vi "Test Asic Rate Scan con tensiones.vi"(8 "Error IN":errorcluster, 11 "Config Test IN":T2={"Config HW"={"VISA Rigol DP832"="Rigol_DP832", "Config Rigol DP832"=[{"Channel"=0, "V Limit"=5.5, "I Limit"=0.5, "V Out"=5.0}, {"Channel"=1, "V Limit"=5.5, "I Limit"=0.8, "V Out"=5.0}, {"Channel"=2, "V Limit"=5.5, "I Limit"=0.2, "V Out"=0.0}], "CTA Test#"="CTA013 A", "FT_Handle"=0, "Espera acceso FT"=10, "VISA Tek MDO3104"="Rigol_DP832", "VISA Key 81160A"="Rigol_DP832"}, "Config Test"=[{"Vasic"=2.8, "Global Reset"=FALSE, "Test Register?"=FALSE, "Test ADC?"=FALSE, "Test ADC"={"Repeats ADC"=100, "Max Desviation"=0.1}, "Limits ADC"={"Low"=[1.9, 1.3, 0.65, 0.0, 1.6, 1.4, 1.4, 0.9, 2.1, 0.85, 1.9], "High"=[2.1, 1.5, 0.85, 0.1, 1.4, 1.2, 1.2, 0.7, 1.9, 0.65, 1.7]}, "Test Max PN Min NP?"=FALSE, "Limits Max PN Min NP"={"Max P Upper"=2.177000045776367, "Min P Upper"=1.474, "Max N Upper"=1.475, "Min N Upper"=0.818, "Max P Lower"=1.888, "Min P Lower "=1.321, "Max N Lower"=1.322, "Min N Lower"=0.73}, "Test Rate Scan?"=FALSE, "Vin Rate Scan"=[], "Limits Rate Scan"={"High"=[0.15, 0.242, 0.331, 0.425, 0.512, 0.6, 0.688, 0.774, 0.847, 0.91], "Low"=[0.021, 0.11, 0.189, 0.27, 0.347, 0.421, 0.487, 0.551, 0.601, 0.635]}, "Test Rate Scan Adders?"=FALSE, "Vin Rate Adders"=[], "Limits Rate Scan adders"={"High"=[], "Low"=[]}, "Test offset analog?"=FALSE, "Lim Offset Analog"={"Max Analog"=0.05, "Min Analog"=-0.05}, "Test offset digital?"=FALSE, "Lim offset Dig"={"Max Dig"=0.05}, "Vasic real f.a."=2.8, "IBIAS"=FALSE, "VALUE IBIAS"=63}, {"Vasic"=2.8, "Global Reset"=FALSE, "Test Register?"=FALSE, "Test ADC?"=FALSE, "Test ADC"={"Repeats ADC"=100, "Max Desviation"=0.1}, "Limits ADC"={"Low"=[1.9, 1.3, 0.65, 0.0, 1.6, 1.4, 1.4, 0.9, 2.1, 0.85, 1.9], "High"=[2.1, 1.5, 0.85, 0.1, 1.4, 1.2, 1.2, 0.7, 1.9, 0.65, 1.7]}, "Test Max PN Min NP?"=FALSE, "Limits Max PN Min NP"={"Max P Upper"=2.177000045776367, "Min P Upper"=1.474, "Max N Upper"=1.475, "Min N Upper"=0.818, "Max P Lower"=1.888, "Min P Lower "=1.321, "Max N Lower"=1.322, "Min N Lower"=0.73}, "Test Rate Scan?"=FALSE, "Vin Rate Scan"=[], "Limits Rate Scan"={"High"=[0.15, 0.242, 0.331, 0.425, 0.512, 0.6, 0.688, 0.774, 0.847, 0.91], "Low"=[0.021, 0.11, 0.189, 0.27, 0.347, 0.421, 0.487, 0.551, 0.601, 0.635]}, "Test Rate Scan Adders?"=FALSE, "Vin Rate Adders"=[], "Limits Rate Scan adders"={"High"=[], "Low"=[]}, "Test offset analog?"=FALSE, "Lim Offset Analog"={"Max Analog"=0.05, "Min Analog"=-0.05}, "Test offset digital?"=FALSE, "Lim offset Dig"={"Max Dig"=0.05}, "Vasic real f.a."=2.8, "IBIAS"=FALSE, "VALUE IBIAS"=63}, {"Vasic"=2.8, "Global Reset"=FALSE, "Test Register?"=FALSE, "Test ADC?"=FALSE, "Test ADC"={"Repeats ADC"=100, "Max Desviation"=0.1}, "Limits ADC"={"Low"=[1.9, 1.3, 0.65, 0.0, 1.6, 1.4, 1.4, 0.9, 2.1, 0.85, 1.9], "High"=[2.1, 1.5, 0.85, 0.1, 1.4, 1.2, 1.2, 0.7, 1.9, 0.65, 1.7]}, "Test Max PN Min NP?"=FALSE, "Limits Max PN Min NP"={"Max P Upper"=2.177000045776367, "Min P Upper"=1.474, "Max N Upper"=1.475, "Min N Upper"=0.818, "Max P Lower"=1.888, "Min P Lower "=1.321, "Max N Lower"=1.322, "Min N Lower"=0.73}, "Test Rate Scan?"=FALSE, "Vin Rate Scan"=[], "Limits Rate Scan"={"High"=[0.15, 0.242, 0.331, 0.425, 0.512, 0.6, 0.688, 0.774, 0.847, 0.91], "Low"=[0.021, 0.11, 0.189, 0.27, 0.347, 0.421, 0.487, 0.551, 0.601, 0.635]}, "Test Rate Scan Adders?"=FALSE, "Vin Rate Adders"=[], "Limits Rate Scan adders"={"High"=[], "Low"=[]}, "Test offset analog?"=FALSE, "Lim Offset Analog"={"Max Analog"=0.05, "Min Analog"=-0.05}, "Test offset digital?"=FALSE, "Lim offset Dig"={"Max Dig"=0.05}, "Vasic real f.a."=2.8, "IBIAS"=FALSE, "VALUE IBIAS"=63}, {"Vasic"=2.8, "Global Reset"=FALSE, "Test Register?"=FALSE, "Test ADC?"=FALSE, "Test ADC"={"Repeats ADC"=100, "Max Desviation"=0.1}, "Limits ADC"={"Low"=[1.9, 1.3, 0.65, 0.0, 1.6, 1.4, 1.4, 0.9, 2.1, 0.85, 1.9], "High"=[2.1, 1.5, 0.85, 0.1, 1.4, 1.2, 1.2, 0.7, 1.9, 0.65, 1.7]}, "Test Max PN Min NP?"=FALSE, "Limits Max PN Min NP"={"Max P Upper"=2.177000045776367, "Min P Upper"=1.474, "Max N Upper"=1.475, "Min N Upper"=0.818, "Max P Lower"=1.888, "Min P Lower "=1.321, "Max N Lower"=1.322, "Min N Lower"=0.73}, "Test Rate Scan?"=FALSE, "Vin Rate Scan"=[], "Limits Rate Scan"={"High"=[0.15, 0.242, 0.331, 0.425, 0.512, 0.6, 0.688, 0.774, 0.847, 0.91], "Low"=[0.021, 0.11, 0.189, 0.27, 0.347, 0.421, 0.487, 0.551, 0.601, 0.635]}, "Test Rate Scan Adders?"=FALSE, "Vin Rate Adders"=[], "Limits Rate Scan adders"={"High"=[], "Low"=[]}, "Test offset analog?"=FALSE, "Lim Offset Analog"={"Max Analog"=0.05, "Min Analog"=-0.05}, "Test offset digital?"=FALSE, "Lim offset Dig"={"Max Dig"=0.05}, "Vasic real f.a."=2.8, "IBIAS"=FALSE, "VALUE IBIAS"=63}], "Result"=[], "Execucion Test"={"Vasic Actual"=0}, "Config VGA"={"Theoretical Voltage"=[], "Real Voltage"=[102.85, 207.14, 299.57, 404.85, 495.71, 606.85, 697.71, 801.14, 897.14, 998.85], "Pulse Width"=57344, "Frecuency Pulse"=1000000.0, "VGA Gain"=[9, 16, 24, 34, 43, 52, 61, 72, 81, 93]}, "Test Info"={"Asic"="", "Operator"="", "Place"="", "Time start"=timestamp(0 s since 1904-01-01), "Time stop"=timestamp(0 s since 1904-01-01)}, "Info machine"={"SO"="", "SO Name"="", "SO Ver"="", "SO Build"="", "CPU"="", "APP"="", "APP YEAR"="", "APP ver"="", "APP User"="", "APP Serail"="", "MAC"=[], "PC NAME"=[], "PC IP"=[], "BIOS MANU"="", "BIOS NAME"="", "BIOS SERIAL"="", "BOARD MANU"="", "BOARD NAME"="", "BOARD SERIAL"="", "Driver Version"="", "Library Version"="", "FPGA Ver"=0, "ID CTA board"=0, "LAST BOOT"="", "LABVIEW Ver"=0}, "Partial Report"="", "CONFIG GEN"=[]} {"CONFIG GEN"."Vasic Theorical" min=1.0 max=1000000.0 step=1.0 format="%#_6pV"; "CONFIG GEN"."Frequency" min=0.001 max=333000000.0 step=1000.0 format="%#_6pHz"; "CONFIG GEN"."Leading Edge Time" min=1e-09 max=1.0 step=1e-10 format="%#_6ps"; "CONFIG GEN"."Trailing Edge Time" min=1e-09 max=1.0 step=1e-10 format="%#_6ps"; "CONFIG GEN"."Delay" min=0.0 max=1.0 step=1e-12 format="%#_6ps"; "CONFIG GEN"."Trigger Level Sync" items=["ECL", "TTL"]; "CONFIG GEN"."Trigger Sync Out" items=["AB"=3, "B"=2, "A"=1, "None"=0]; "CONFIG GEN"."Load" min=1.0 max=1000000.0 step=1.0 format="%#_6p"; "CONFIG GEN"."DC Offset" min=-10.0 max=10.0 step=0.1 format="%#_6pV"; "CONFIG GEN"."Amplitude" min=0.05 max=5.0 step=0.001 format="%#_6pV"; "CONFIG GEN"."Width Time" min=1.5e-09 max=1.0 step=1e-10 format="%#_6ps"; "CONFIG GEN"."Channel" items=["Channel1"=1, "Channel2"=2]; "Config VGA"."Theoretical Voltage" format="%1.4f"; "Config VGA"."VGA Gain" format="%02x"; "Config VGA"."Frecuency Pulse" format="%0_2p"; "Config VGA"."Pulse Width" format="%04x"; "Config VGA"."Real Voltage" format="%1.5f"; "Config Test"."VALUE IBIAS" max=63 step=1; "Config Test"."Vasic real f.a." min=2.8 max=3.8 step=0.01 format="%.2g"; "Config Test"."Limits Rate Scan adders"."Low" format="%1.3f"; "Config Test"."Limits Rate Scan adders"."High" format="%1.3f"; "Config Test"."Limits ADC"."High" format="%1.4f"; "Config Test"."Limits ADC"."Low" format="%1.3f"; "Config Test"."Lim offset Dig"."Max Dig" format="%.3g"; "Config Test"."Lim Offset Analog"."Min Analog" format="%.3g"; "Config Test"."Lim Offset Analog"."Max Analog" format="%.3g"; "Config Test"."Limits Rate Scan"."Low" format="%1.4f"; "Config Test"."Limits Rate Scan"."High" format="%1.3f"; "Config Test"."Limits Max PN Min NP"."Min P Upper" format="%.3g"; "Config Test"."Limits Max PN Min NP"."Min P Lower" format="%.3g"; "Config Test"."Limits Max PN Min NP"."Max N Lower" format="%.3g"; "Config Test"."Limits Max PN Min NP"."Max N Upper" format="%.3g"; "Config Test"."Limits Max PN Min NP"."Min N Lower" format="%.3g"; "Config Test"."Limits Max PN Min NP"."Min N Upper" format="%.3g"; "Config Test"."Limits Max PN Min NP"."Max P Upper" format="%.3g"; "Config Test"."Limits Max PN Min NP"."Max P Lower" format="%.3g"; "Config Test"."Vasic" min=2.8 max=3.8 step=0.01 format="%.2g"; "Config HW"."Config Rigol DP832"."Channel" items=["+30V Channel 1", "+30V Channel 2", "+5V Channel 3"]; "Config HW"."Config Rigol DP832"."V Limit" format="%.1g"; "Config HW"."Config Rigol DP832"."I Limit" format="%.1g"; "Config HW"."Config Rigol DP832"."V Out" format="%.1g"; "Result"."Test Registros"."Read W/R" format="%04x"; "Result"."Test Registros"."Pattern W/R" format="%04x"; "Result"."Test Registros"."Read Default" format="%04x"; "Result"."Test Registros"."Pattern Default" format="%04x"}) -> (0 "Error OUT":errorcluster, 2 "Rate scan all ok":bool, 3 "Config Test OUT":T2={"Config HW"={"VISA Rigol DP832"="Rigol_DP832", "Config Rigol DP832"=[{"Channel"=0, "V Limit"=5.5, "I Limit"=0.5, "V Out"=5.0}, {"Channel"=1, "V Limit"=5.5, "I Limit"=0.8, "V Out"=5.0}, {"Channel"=2, "V Limit"=5.5, "I Limit"=0.2, "V Out"=0.0}], "CTA Test#"="CTA013 A", "FT_Handle"=0, "Espera acceso FT"=10, "VISA Tek MDO3104"="Rigol_DP832", "VISA Key 81160A"="Rigol_DP832"}, "Config Test"=[{"Vasic"=2.8, "Global Reset"=FALSE, "Test Register?"=FALSE, "Test ADC?"=FALSE, "Test ADC"={"Repeats ADC"=100, "Max Desviation"=0.1}, "Limits ADC"={"Low"=[1.9, 1.3, 0.65, 0.0, 1.6, 1.4, 1.4, 0.9, 2.1, 0.85, 1.9], "High"=[2.1, 1.5, 0.85, 0.1, 1.4, 1.2, 1.2, 0.7, 1.9, 0.65, 1.7]}, "Test Max PN Min NP?"=FALSE, "Limits Max PN Min NP"={"Max P Upper"=2.177000045776367, "Min P Upper"=1.474, "Max N Upper"=1.475, "Min N Upper"=0.818, "Max P Lower"=1.888, "Min P Lower "=1.321, "Max N Lower"=1.322, "Min N Lower"=0.73}, "Test Rate Scan?"=FALSE, "Vin Rate Scan"=[], "Limits Rate Scan"={"High"=[0.15, 0.242, 0.331, 0.425, 0.512, 0.6, 0.688, 0.774, 0.847, 0.91], "Low"=[0.021, 0.11, 0.189, 0.27, 0.347, 0.421, 0.487, 0.551, 0.601, 0.635]}, "Test Rate Scan Adders?"=FALSE, "Vin Rate Adders"=[], "Limits Rate Scan adders"={"High"=[], "Low"=[]}, "Test offset analog?"=FALSE, "Lim Offset Analog"={"Max Analog"=0.05, "Min Analog"=-0.05}, "Test offset digital?"=FALSE, "Lim offset Dig"={"Max Dig"=0.05}, "Vasic real f.a."=2.8, "IBIAS"=FALSE, "VALUE IBIAS"=63}, {"Vasic"=2.8, "Global Reset"=FALSE, "Test Register?"=FALSE, "Test ADC?"=FALSE, "Test ADC"={"Repeats ADC"=100, "Max Desviation"=0.1}, "Limits ADC"={"Low"=[1.9, 1.3, 0.65, 0.0, 1.6, 1.4, 1.4, 0.9, 2.1, 0.85, 1.9], "High"=[2.1, 1.5, 0.85, 0.1, 1.4, 1.2, 1.2, 0.7, 1.9, 0.65, 1.7]}, "Test Max PN Min NP?"=FALSE, "Limits Max PN Min NP"={"Max P Upper"=2.177000045776367, "Min P Upper"=1.474, "Max N Upper"=1.475, "Min N Upper"=0.818, "Max P Lower"=1.888, "Min P Lower "=1.321, "Max N Lower"=1.322, "Min N Lower"=0.73}, "Test Rate Scan?"=FALSE, "Vin Rate Scan"=[], "Limits Rate Scan"={"High"=[0.15, 0.242, 0.331, 0.425, 0.512, 0.6, 0.688, 0.774, 0.847, 0.91], "Low"=[0.021, 0.11, 0.189, 0.27, 0.347, 0.421, 0.487, 0.551, 0.601, 0.635]}, "Test Rate Scan Adders?"=FALSE, "Vin Rate Adders"=[], "Limits Rate Scan adders"={"High"=[], "Low"=[]}, "Test offset analog?"=FALSE, "Lim Offset Analog"={"Max Analog"=0.05, "Min Analog"=-0.05}, "Test offset digital?"=FALSE, "Lim offset Dig"={"Max Dig"=0.05}, "Vasic real f.a."=2.8, "IBIAS"=FALSE, "VALUE IBIAS"=63}, {"Vasic"=2.8, "Global Reset"=FALSE, "Test Register?"=FALSE, "Test ADC?"=FALSE, "Test ADC"={"Repeats ADC"=100, "Max Desviation"=0.1}, "Limits ADC"={"Low"=[1.9, 1.3, 0.65, 0.0, 1.6, 1.4, 1.4, 0.9, 2.1, 0.85, 1.9], "High"=[2.1, 1.5, 0.85, 0.1, 1.4, 1.2, 1.2, 0.7, 1.9, 0.65, 1.7]}, "Test Max PN Min NP?"=FALSE, "Limits Max PN Min NP"={"Max P Upper"=2.177000045776367, "Min P Upper"=1.474, "Max N Upper"=1.475, "Min N Upper"=0.818, "Max P Lower"=1.888, "Min P Lower "=1.321, "Max N Lower"=1.322, "Min N Lower"=0.73}, "Test Rate Scan?"=FALSE, "Vin Rate Scan"=[], "Limits Rate Scan"={"High"=[0.15, 0.242, 0.331, 0.425, 0.512, 0.6, 0.688, 0.774, 0.847, 0.91], "Low"=[0.021, 0.11, 0.189, 0.27, 0.347, 0.421, 0.487, 0.551, 0.601, 0.635]}, "Test Rate Scan Adders?"=FALSE, "Vin Rate Adders"=[], "Limits Rate Scan adders"={"High"=[], "Low"=[]}, "Test offset analog?"=FALSE, "Lim Offset Analog"={"Max Analog"=0.05, "Min Analog"=-0.05}, "Test offset digital?"=FALSE, "Lim offset Dig"={"Max Dig"=0.05}, "Vasic real f.a."=2.8, "IBIAS"=FALSE, "VALUE IBIAS"=63}, {"Vasic"=2.8, "Global Reset"=FALSE, "Test Register?"=FALSE, "Test ADC?"=FALSE, "Test ADC"={"Repeats ADC"=100, "Max Desviation"=0.1}, "Limits ADC"={"Low"=[1.9, 1.3, 0.65, 0.0, 1.6, 1.4, 1.4, 0.9, 2.1, 0.85, 1.9], "High"=[2.1, 1.5, 0.85, 0.1, 1.4, 1.2, 1.2, 0.7, 1.9, 0.65, 1.7]}, "Test Max PN Min NP?"=FALSE, "Limits Max PN Min NP"={"Max P Upper"=2.177000045776367, "Min P Upper"=1.474, "Max N Upper"=1.475, "Min N Upper"=0.818, "Max P Lower"=1.888, "Min P Lower "=1.321, "Max N Lower"=1.322, "Min N Lower"=0.73}, "Test Rate Scan?"=FALSE, "Vin Rate Scan"=[], "Limits Rate Scan"={"High"=[0.15, 0.242, 0.331, 0.425, 0.512, 0.6, 0.688, 0.774, 0.847, 0.91], "Low"=[0.021, 0.11, 0.189, 0.27, 0.347, 0.421, 0.487, 0.551, 0.601, 0.635]}, "Test Rate Scan Adders?"=FALSE, "Vin Rate Adders"=[], "Limits Rate Scan adders"={"High"=[], "Low"=[]}, "Test offset analog?"=FALSE, "Lim Offset Analog"={"Max Analog"=0.05, "Min Analog"=-0.05}, "Test offset digital?"=FALSE, "Lim offset Dig"={"Max Dig"=0.05}, "Vasic real f.a."=2.8, "IBIAS"=FALSE, "VALUE IBIAS"=63}], "Result"=[], "Execucion Test"={"Vasic Actual"=0}, "Config VGA"={"Theoretical Voltage"=[], "Real Voltage"=[102.85, 207.14, 299.57, 404.85, 495.71, 606.85, 697.71, 801.14, 897.14, 998.85], "Pulse Width"=57344, "Frecuency Pulse"=1000000.0, "VGA Gain"=[9, 16, 24, 34, 43, 52, 61, 72, 81, 93]}, "Test Info"={"Asic"="", "Operator"="", "Place"="", "Time start"=timestamp(0 s since 1904-01-01), "Time stop"=timestamp(0 s since 1904-01-01)}, "Info machine"={"SO"="", "SO Name"="", "SO Ver"="", "SO Build"="", "CPU"="", "APP"="", "APP YEAR"="", "APP ver"="", "APP User"="", "APP Serail"="", "MAC"=[], "PC NAME"=[], "PC IP"=[], "BIOS MANU"="", "BIOS NAME"="", "BIOS SERIAL"="", "BOARD MANU"="", "BOARD NAME"="", "BOARD SERIAL"="", "Driver Version"="", "Library Version"="", "FPGA Ver"=0, "ID CTA board"=0, "LAST BOOT"="", "LABVIEW Ver"=0}, "Partial Report"="", "CONFIG GEN"=[]} {"CONFIG GEN"."Vasic Theorical" min=1.0 max=1000000.0 step=1.0 format="%#_6pV"; "CONFIG GEN"."Frequency" min=0.001 max=333000000.0 step=1000.0 format="%#_6pHz"; "CONFIG GEN"."Leading Edge Time" min=1e-09 max=1.0 step=1e-10 format="%#_6ps"; "CONFIG GEN"."Trailing Edge Time" min=1e-09 max=1.0 step=1e-10 format="%#_6ps"; "CONFIG GEN"."Delay" min=0.0 max=1.0 step=1e-12 format="%#_6ps"; "CONFIG GEN"."Trigger Level Sync" items=["ECL", "TTL"]; "CONFIG GEN"."Trigger Sync Out" items=["AB"=3, "B"=2, "A"=1, "None"=0]; "CONFIG GEN"."Load" min=1.0 max=1000000.0 step=1.0 format="%#_6p"; "CONFIG GEN"."DC Offset" min=-10.0 max=10.0 step=0.1 format="%#_6pV"; "CONFIG GEN"."Amplitude" min=0.05 max=5.0 step=0.001 format="%#_6pV"; "CONFIG GEN"."Width Time" min=1.5e-09 max=1.0 step=1e-10 format="%#_6ps"; "CONFIG GEN"."Channel" items=["Channel1"=1, "Channel2"=2]; "Config VGA"."Theoretical Voltage" format="%1.4f"; "Config VGA"."VGA Gain" format="%02x"; "Config VGA"."Frecuency Pulse" format="%0_2p"; "Config VGA"."Pulse Width" format="%04x"; "Config VGA"."Real Voltage" format="%1.5f"; "Config Test"."VALUE IBIAS" max=63 step=1; "Config Test"."Vasic real f.a." min=2.8 max=3.8 step=0.01 format="%.2g"; "Config Test"."Limits Rate Scan adders"."Low" format="%1.3f"; "Config Test"."Limits Rate Scan adders"."High" format="%1.3f"; "Config Test"."Limits ADC"."High" format="%1.4f"; "Config Test"."Limits ADC"."Low" format="%1.3f"; "Config Test"."Lim offset Dig"."Max Dig" format="%.3g"; "Config Test"."Lim Offset Analog"."Min Analog" format="%.3g"; "Config Test"."Lim Offset Analog"."Max Analog" format="%.3g"; "Config Test"."Limits Rate Scan"."Low" format="%1.4f"; "Config Test"."Limits Rate Scan"."High" format="%1.3f"; "Config Test"."Limits Max PN Min NP"."Min P Upper" format="%.3g"; "Config Test"."Limits Max PN Min NP"."Min P Lower" format="%.3g"; "Config Test"."Limits Max PN Min NP"."Max N Lower" format="%.3g"; "Config Test"."Limits Max PN Min NP"."Max N Upper" format="%.3g"; "Config Test"."Limits Max PN Min NP"."Min N Lower" format="%.3g"; "Config Test"."Limits Max PN Min NP"."Min N Upper" format="%.3g"; "Config Test"."Limits Max PN Min NP"."Max P Upper" format="%.3g"; "Config Test"."Limits Max PN Min NP"."Max P Lower" format="%.3g"; "Config Test"."Vasic" min=2.8 max=3.8 step=0.01 format="%.2g"; "Config HW"."Config Rigol DP832"."Channel" items=["+30V Channel 1", "+30V Channel 2", "+5V Channel 3"]; "Config HW"."Config Rigol DP832"."V Limit" format="%.1g"; "Config HW"."Config Rigol DP832"."I Limit" format="%.1g"; "Config HW"."Config Rigol DP832"."V Out" format="%.1g"; "Result"."Test Registros"."Read W/R" format="%04x"; "Result"."Test Registros"."Pattern W/R" format="%04x"; "Result"."Test Registros"."Read Default" format="%04x"; "Result"."Test Registros"."Pattern Default" format="%04x"})   [LabVIEW 2019]
uses:
  Test.ctl
  TEST.TEST CONFIG HW.ctl
  Rigol DP832/DP832_Control Channels.ctl
  TEST.TEST CONFIG TEST MATRIZ.ctl
  TEST.TEST CONFIG TEST.ctl
  TEST.TEST RESULT.ctl
  test_result fvasic.ctl
  TEST.TEST EXECUTION TEST.ctl
  TEST.TEST CONFIG VGA.ctl
  TEST.TEST TEST INFO.ctl
  TEST.TEST INFO PC.ctl
  GenPulse_configurar.ctl
  Global.Salir Ya.vi
panel:
  out "Array 2":dbl[](array[numeric])
  out "Array":dbl[](array[numeric])
  in  "DAC\nTH0,TH1,TH2":u16
  in  "Tab Control":enum32{"Page 1", "Page 2"}(tab)
  out "%":u8 format="%02d%%"
  out "B":u8(slide) scale=0.0..100.0
  out "Indicador":string
  out "Comparation LLTH":bool[][][](array[boolean])
  out "Comparation HLTH":bool[][][](array[boolean])
  out "Reference":T1
  out "DAC TH3,TH4,TH5":u16
  out "LLTHx":dbl
  out "DAC TH0,TH1,TH2":u16
  out "HLTHx":dbl
  out "Volt LLTH (salida B)":dbl[][][](array[numeric])
  out "Volt HLTH (salida A)":dbl[][][](array[numeric])
  out "DAC TH3,TH4,TH5":u16[][][](array[numeric])
  out "DAC TH0,TH1,TH2":u16[][][](array[numeric])
  # "Vin Asic"
  # "Canal"
  # "Sumador"
  # "Test ASIC. Rate Scan"
  # "Modo 2\nModo 3\nModo 4\nModo 2\nModo 3\nModo 4"
  # "Modo 2\nModo 3\nModo 4\nModo 2\nModo 3\nModo 4"
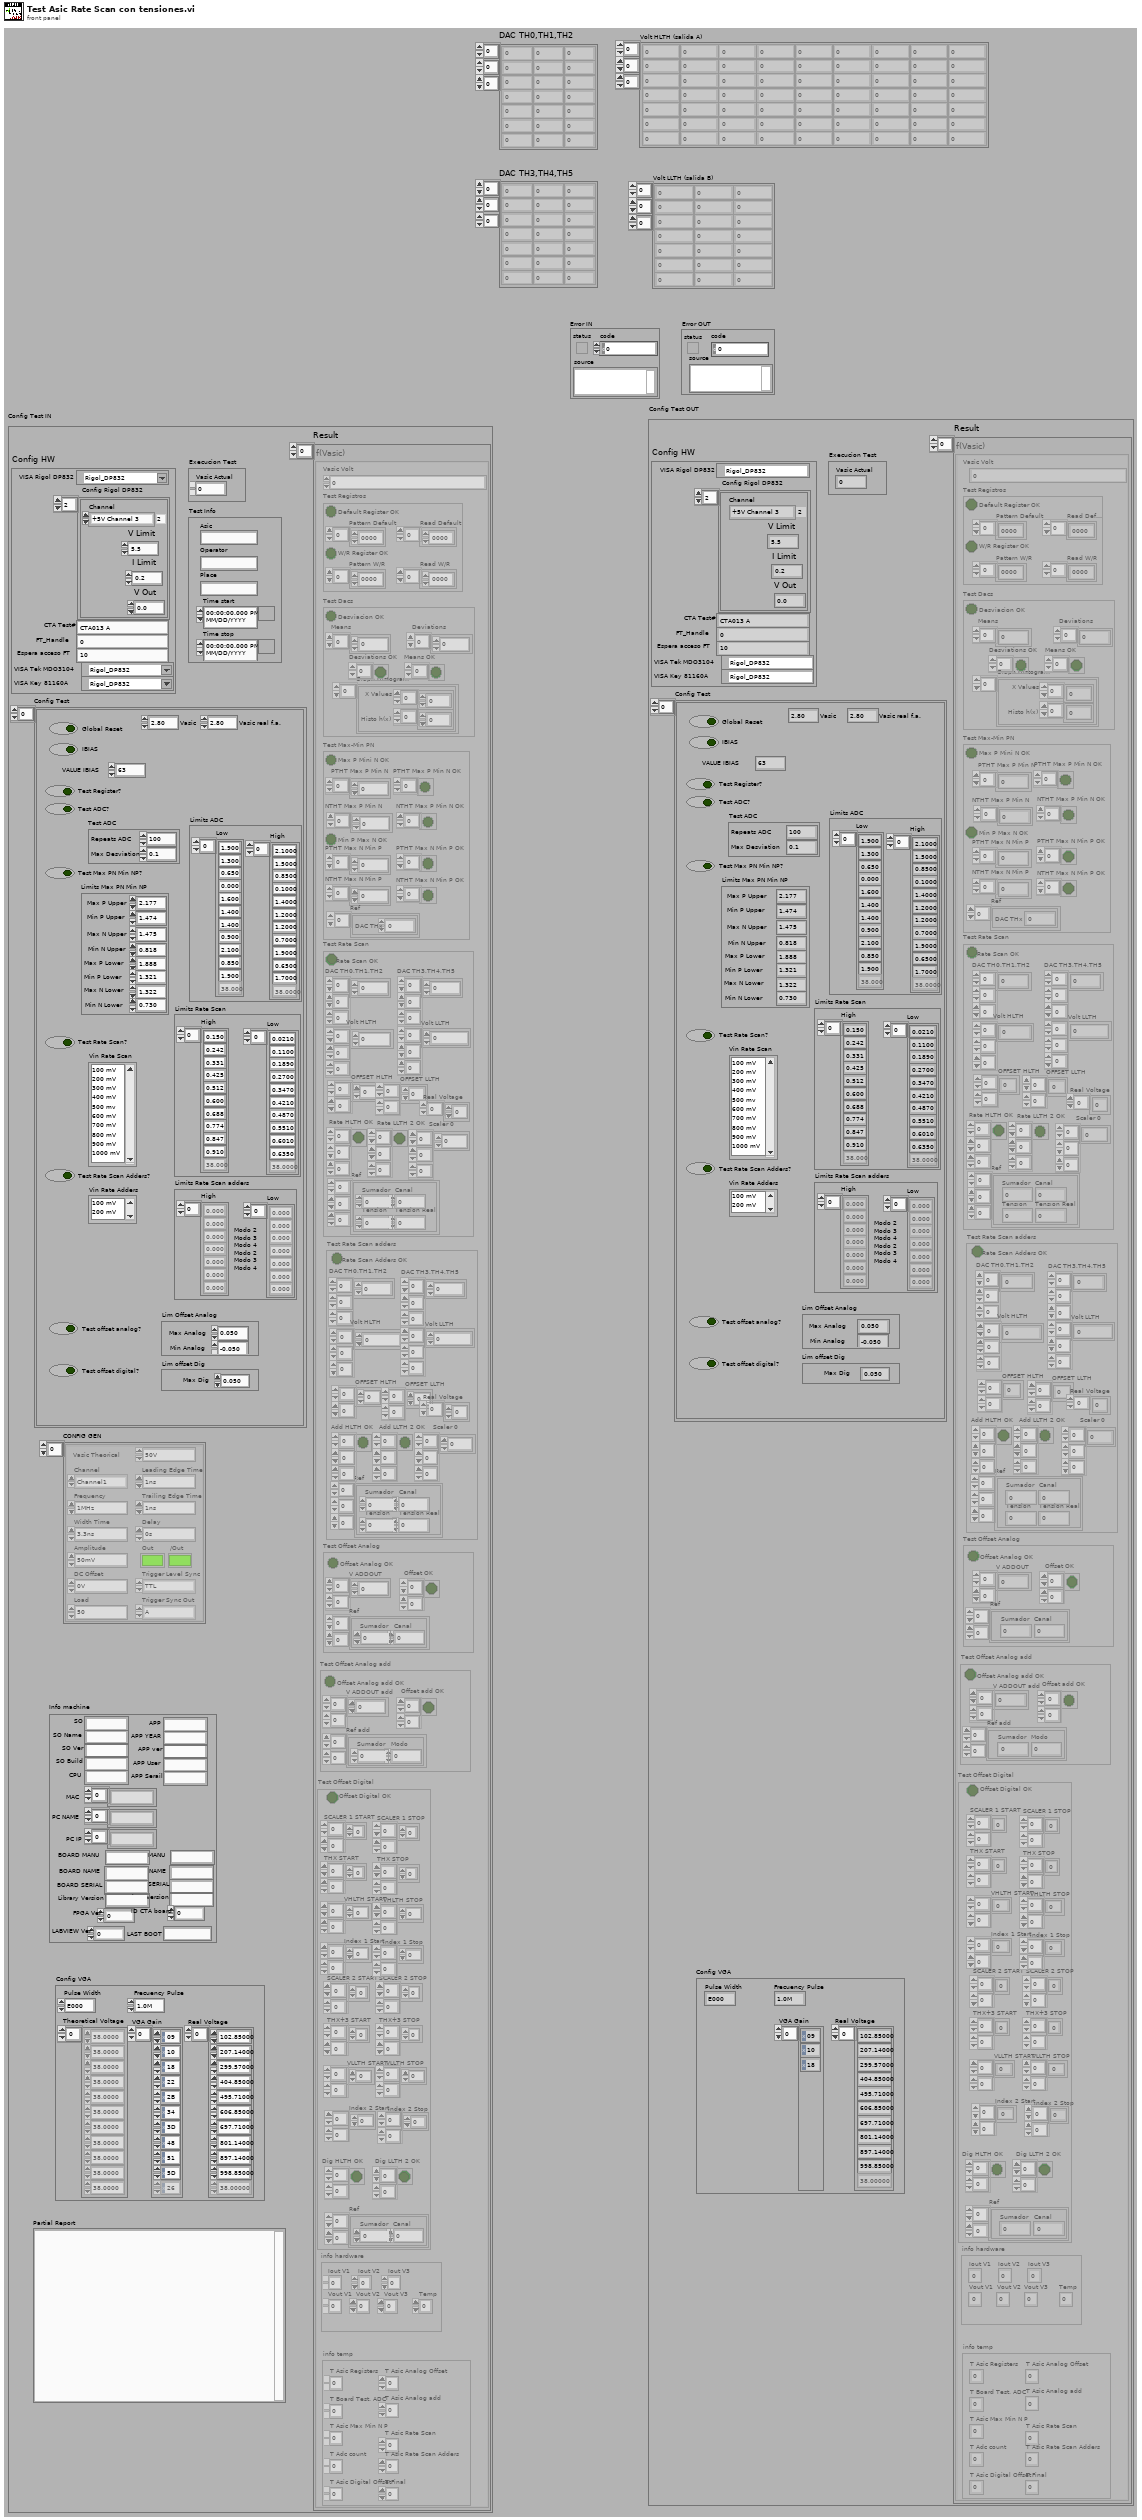
[diagram p1: front panel]
types:
  T1 = cluster{"Sumador":u8, "Canal":u8, "Tension":u8, "Tension Real":dbl}
  T2 = typedef "Test.ctl" = cluster{"Config HW":T3, "Config Test":T5, "Result":T7, "Execucion Test":T9, "Config VGA":T10, "Test Info":T11, "Info machine":T12, "Partial Report":string, "CONFIG GEN":T13[]}
  T3 = typedef "TEST.TEST CONFIG HW.ctl" = cluster{"VISA Rigol DP832":refnum<visa-resource-name>, "Config Rigol DP832":cluster{"Channel":T4, "V Limit":dbl, "I Limit":dbl, "V Out":dbl}[], "CTA Test#":string, "FT_Handle":u32, "Espera acceso FT":u32, "VISA Tek MDO3104":refnum<visa-resource-name>, "VISA Key 81160A":refnum<visa-resource-name>}
  T4 = typedef "DP832_Control Channels.ctl" = i32
  T5 = typedef "TEST.TEST CONFIG TEST MATRIZ.ctl" = T6[]
  T6 = typedef "TEST.TEST CONFIG TEST.ctl" = cluster{"Vasic":dbl, "Global Reset":bool, "Test Register?":bool, "Test ADC?":bool, "Test ADC":cluster{"Repeats ADC":i32, "Max Desviation":dbl}, "Limits ADC":cluster{"Low":dbl[], "High":dbl[]}, "Test Max PN Min NP?":bool, "Limits Max PN Min NP":cluster{"Max P Upper":dbl, "Min P Upper":dbl, "Max N Upper":dbl, "Min N Upper":dbl, "Max P Lower":dbl, "Min P Lower ":dbl, "Max N Lower":dbl, "Min N Lower":dbl}, "Test Rate Scan?":bool, "Vin Rate Scan":i32[], "Limits Rate Scan":cluster{"High":dbl[], "Low":dbl[]}, "Test Rate Scan Adders?":bool, "Vin Rate Adders":i32[], "Limits Rate Scan adders":cluster{"High":dbl[], "Low":dbl[]}, "Test offset analog?":bool, "Lim Offset Analog":cluster{"Max Analog":dbl, "Min Analog":dbl}, "Test offset digital?":bool, "Lim offset Dig":cluster{"Max Dig":dbl}, "Vasic real f.a.":dbl, "IBIAS":bool, "VALUE IBIAS":u8}
  T7 = typedef "TEST.TEST RESULT.ctl" = T8[]
  T8 = typedef "test_result fvasic.ctl" = cluster{"Vasic Volt":i32, "Test Registros":cluster{"Default Register OK":bool, "Pattern Default":u16[], "Read Default":u16[], "W/R Register OK":bool, "Pattern W/R":u16[], "Read W/R":u16[]}, "Test Dacs":cluster{"Desviacion OK":bool, "Means":dbl[], "Deviations":dbl[], "Desviations OK":bool[], "Means OK":bool[], "Graph Histogram":cluster{"X Values":dbl[], "Histo h(x)":i32[]}[]}, "Test Max-Min PN":cluster{"Max P Mini N OK":bool, "PTHT Max P Min N":dbl[], "PTHT Max P Min N OK":bool[], "NTHT Max P Min N":dbl[], "NTHT Max P Min N OK":bool[], "Min P Max N OK":bool, "PTHT Max N Min P":dbl[], "PTHT Max N Min P OK":bool[], "NTHT Max N Min P":dbl[], "NTHT Max N Min P OK":bool[], "Ref":cluster{"DAC THx":u8}[]}, "Test Rate Scan":cluster{"Rate Scan OK":bool, "DAC TH0,TH1,TH2":u16[][][], "Volt HLTH":dbl[][][], "Rate HLTH OK":bool[][][], "DAC TH3,TH4,TH5":u16[][][], "Volt LLTH":dbl[][][], "Rate LLTH 2 OK":bool[][][], "Scaler 0":u16[][][], "Ref":cluster{"Sumador":u8, "Canal":u8, "Tension":u8, "Tension Real":dbl}[][][], "OFFSET HLTH":dbl[][], "OFFSET LLTH":dbl[][], "Real Voltage":dbl[]}, "Test Rate Scan adders":cluster{"Rate Scan Adders OK":bool, "DAC TH0,TH1,TH2":u16[][][], "Volt HLTH":dbl[][][], "Add HLTH OK":bool[][][], "DAC TH3,TH4,TH5":u16[][][], "Volt LLTH":dbl[][][], "Add LLTH 2 OK":bool[][][], "Scaler 0":u16[][][], "Ref":cluster{"Sumador":u8, "Canal":u8, "Tension":u8, "Tension Real":dbl}[][][], "OFFSET HLTH":dbl[][], "OFFSET LLTH":dbl[][], "Real Voltage":dbl[]}, "Test Offset Analog":cluster{"Offset Analog OK":bool, "V ADDOUT":dbl[][], "Offset OK":bool[][], "Ref":cluster{"Sumador":u8, "Canal":u8}[][]}, "Test Offset Digital":cluster{"Offset Digital OK":bool, "SCALER 1 START":u16[][], "SCALER 1 STOP":u16[][], "THX START":u16[][], "THX STOP":u16[][], "VHLTH START":dbl[][], "VHLTH STOP":dbl[][], "Index 1 Start":i32[][], "index 1 Stop":i32[][], "SCALER 2 START":u16[][], "SCALER 2 STOP":u16[][], "THX+3 START":u16[][], "THX+3 STOP":u16[][], "VLLTH START":dbl[][], "VLLTH STOP":dbl[][], "Index 2 Start":i32[][], "index 2 Stop":i32[][], "Dig HLTH OK":bool[][], "Dig LLTH 2 OK":bool[][], "Ref":cluster{"Sumador":u8, "Canal":u8}[][]}, "info hardware":cluster{"Iout V1":dbl, "Iout V2":dbl, "Iout V3":dbl, "Vout V1":dbl, "Vout V2":dbl, "Vout V3":dbl, "Temp":dbl}, "Test Offset Analog add":cluster{"Offset Analog add OK":bool, "V ADDOUT add":dbl[][], "Offset add OK":bool[][], "Ref add":cluster{"Sumador":u8, "Modo":u8}[][]}, "info temp":cluster{"T Asic Registers":dbl, "T Board Test. ADC":dbl, "T Asic Max Min N P":dbl, "T Adc count":dbl, "T Asic Digital Offset":dbl, "T Asic Analog Offset":dbl, "T Asic Analog add":dbl, "T Asic Rate Scan":dbl, "T Asic Rate Scan Adders":dbl, "T Final":dbl}}
  T9 = typedef "TEST.TEST EXECUTION TEST.ctl" = cluster{"Vasic Actual":i32}
  T10 = typedef "TEST.TEST CONFIG VGA.ctl" = cluster{"Theoretical Voltage":dbl[], "Real Voltage":dbl[], "Pulse Width":u16, "Frecuency Pulse":dbl, "VGA Gain":u8[]}
  T11 = typedef "TEST.TEST TEST INFO.ctl" = cluster{"Asic":string, "Operator":string, "Place":string, "Time start":timestamp, "Time stop":timestamp}
  T12 = typedef "TEST.TEST INFO PC.ctl" = cluster{"SO":string, "SO Name":string, "SO Ver":string, "SO Build":string, "CPU":string, "APP":string, "APP YEAR":string, "APP ver":string, "APP User":string, "APP Serail":string, "MAC":string[], "PC NAME":string[], "PC IP":string[], "BIOS MANU":string, "BIOS NAME":string, "BIOS SERIAL":string, "BOARD MANU":string, "BOARD NAME":string, "BOARD SERIAL":string, "Driver Version":string, "Library Version":string, "FPGA Ver":u8, "ID CTA board":u64, "LAST BOOT":string, "LABVIEW Ver":u32}
  T13 = typedef "GenPulse_configurar.ctl" = cluster{"Channel":u16, "Frequency":dbl, "Width Time":dbl, "Amplitude":dbl, "DC Offset":dbl, "Load":dbl, "Leading Edge Time":dbl, "Trailing Edge Time":dbl, "Delay":dbl, "Out":bool, "/Out":bool, "Trigger Level Sync":u16, "Trigger Sync Out":u16, "Vasic Theorical":dbl}
  T14 = enum16{"Always On", "Always Off", "Off While Running"}
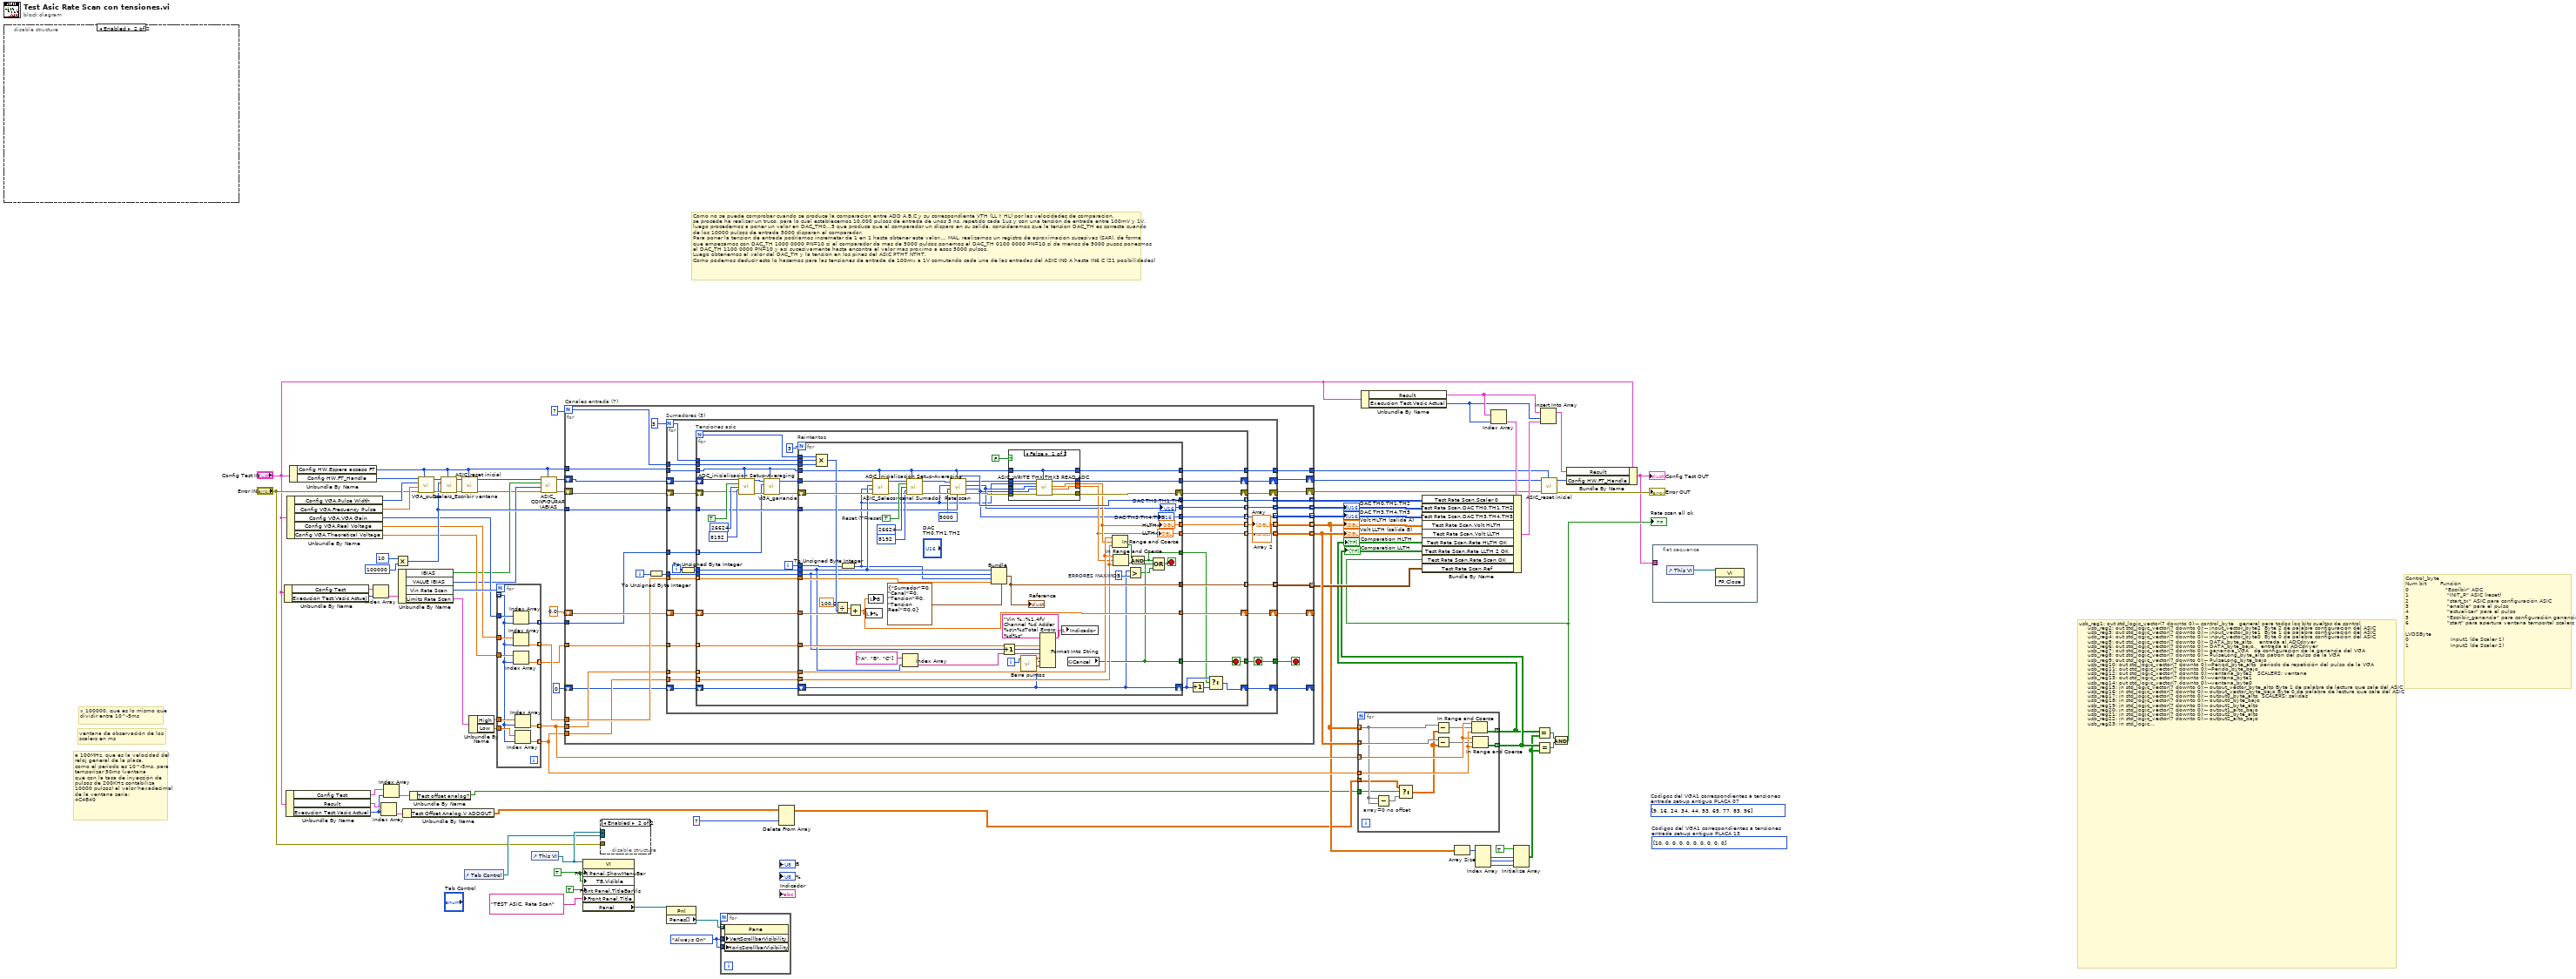
[diagram p0: block diagram]
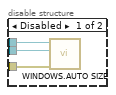
[diagram p2: hidden frame]
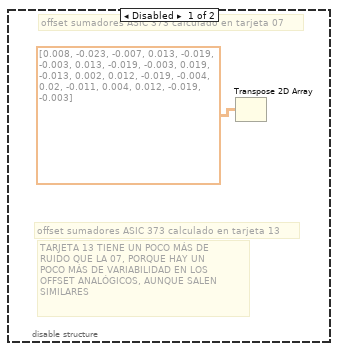
[diagram p3: hidden frame]
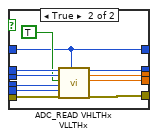
[diagram p4: hidden frame]
diagram:
  w1 = T14."Always On" ("Vertical Scrollbar Visibility")
  w35 = TRUE ("Front Panel Window:Show Menu Bar")
  (unwired) u8[] [10, 0, 0, 0, 0, 0, 0, 0, 0, 0]  # Códigos del VGA1 correspondientes a tensiones entrada set-up antiguo PLACA 13
  (unwired) u8[] [9, 16, 24, 34, 44, 53, 65, 77, 83, 96]  # Códigos del VGA1 correspondientes a tensiones entrada set-up antiguo PLACA 07
  # "Como no se puede comprobar cuando se produce la comparacion entre ADD A,B,C y su correspondiente VTH (LL Y HL) por las velocidades de comparacion,\nse procede ha realizar un truco, para lo cual establecemos 10.000 pulsos de entrada de unos 3 ns, repetido cada 1us y con una tension de entrada entre 100mV y 1V,\nluego procedemos a poner un valor en DAC_TH0...5 que produca que el comparador un disparo en su salida, consideramos que la tension DAC_TH es correcta cuando\nde los 10000 pulsos de entrada 5000 disparan el comparador.\nPara poner la tension de entrada podriamos incremetar de 1 en 1 hasta obtener este valor.... MAL. realizamos un registro de aproximacion sucesivas (SAR), de forma\nque empezamos con DAC_TH 1000 0000 PN=10 si el comparador da mas de 5000 pulsos ponemos el DAC_TH 0100 0000 PN=10 si da menos de 5000 pusos ponesmos\nel DAC_TH 1100 0000 PN=10 y asi sucesivamente hasta encontra el valor mas proximo a esos 5000 pulsos. \nLuego obtenemos el valor del DAC_TH y la tension en los pines del ASIC PTHT NTHT.\nComo podemos deducir esto lo hacemos para las tensiones de entrada de 100mv a 1V comutando cada una de las entradas del ASIC IN0 A hasta IN6 C (21 posibilidades)"
  # "Control_byte\nNum bit        Función\n0                     \"Escribir\" ADC\n1                      \"INIT_R\" ASIC (reset)\n2                      \"start_tx\" ASIC para configuración ASIC\n3                      \"enable\" para el pulso\n4                      \"actualizar\" para el pulso\n5                      \"Escribir_ganancia\" para configuración ganancia\n6                      \"start\" para apertura ventana temportal scalers\n\nLVDSByte\n0                        Input1 (de Scaler 1)\n1                        Input2 (de Scaler 2)"
  # "usb_reg1: out std_logic_vector(7 downto 0);-- control_byte\t\t\tgeneral para todos los bits sueltos de control\n\t\t\t  usb_reg2: out std_logic_vector(7 downto 0);-- input_vector_byte2 \tByte 2 de palabra configuración del ASIC\n\t\t\t  usb_reg3: out std_logic_vector(7 downto 0);-- input_vector_byte1 \tByte 1 de palabra configuración del ASIC\n\t\t\t  usb_reg4: out std_logic_vector(7 downto 0);-- input_vector_byte0 \tByte 0 de palabra configuración del ASIC\n\t\t\t  usb_reg5: out std_logic_vector(7 downto 0);-- DATA_byte_alto, \t\tentrada al ADCdriver\n\t\t\t  usb_reg6: out std_logic_vector(7 downto 0);-- DATA_byte_bajo, \t\tentrada al ADCdriver\n\t\t\t  usb_reg7: out std_logic_vector(7 downto 0);-- ganancia_VGA\t\t\tde configuración de la ganancia del VGA\n\t\t\t  usb_reg8: out std_logic_vector(7 downto 0);-- PulseLong_byte_alto\tpatrón del pulso de la VGA\n\t\t\t  usb_reg9: out std_logic_vector(7 downto 0);-- PulseLong_byte_bajo\n\t\t\t  usb_reg10: out std_logic_vector(7 downto 0);--Period_byte_alto\t\tperíodo de repetición del pulso de la VGA\n\t\t\t  usb_reg11: out std_logic_vector(7 downto 0);--Perido_byte_bajo\n\t\t\t  usb_reg12: out std_logic_vector(7 downto 0);--ventana_byte2\t\t\tSCALERS: ventana\n\t\t\t  usb_reg13: out std_logic_vector(7 downto 0);--ventana_byte1\t\n\t\t\t  usb_reg14: out std_logic_vector(7 downto 0);--ventana_byte0\n\t\t\t  usb_reg15: in std_logic_vector(7 downto 0);-- output_vector_byte_alto\tByte 1 de palabra de lectura que sale del ASIC\n\t\t\t  usb_reg16: in std_logic_vector(7 downto 0);-- output_vector_byte_bajo\tByte 0 de palabra de lectura que sale del ASIC\n\t\t\t  usb_reg17: in std_logic_vector(7 downto 0);-- output0_byte_alto\t\tSCALERS: salidas\n\t\t\t  usb_reg18: in std_logic_vector(7 downto 0);-- output0_byte_bajo\n\t\t\t  usb_reg19: in std_logic_vector(7 downto 0);-- output1_byte_alto\n\t\t\t  usb_reg20: in std_logic_vector(7 downto 0);-- output1_alto_bajo \n\t\t\t  usb_reg21: in std_logic_vector(7 downto 0);-- output2_byte_alto \n\t\t\t  usb_reg22: in std_logic_vector(7 downto 0);-- output2_alto_bajo \n\t\t\t  usb_reg23: in std_logic_vector(7 downto 0);-- para el canal_0 del ADCdriver\n\t\t\t  usb_reg24: in std_logic_vector(7 downto 0);\n\t\t\t  usb_reg25: in std_logic_vector(7 downto 0);-- para el canal_1 del ADCdriver\n\t\t\t  usb_reg26: in std_logic_vector(7 downto 0);\n\t\t\t  usb_reg27: in std_logic_vector(7 downto 0);-- para el canal_2 del ADCdriver\n\t\t\t  usb_reg28: in std_logic_vector(7 downto 0);\n\t\t\t  usb_reg29: in std_logic_vector(7 downto 0);-- para el canal_3 del ADCdriver\n\t\t\t  usb_reg30: in std_logic_vector(7 downto 0);\n\t\t\t  usb_reg31: in std_logic_vector(7 downto 0);-- para el canal_4 del ADCdriver\n\t\t\t  usb_reg32: in std_logic_vector(7 downto 0);\n\t\t\t  usb_reg33: in std_logic_vector(7 downto 0);-- para el canal_5 del ADCdriver\n\t\t\t  usb_reg34: in std_logic_vector(7 downto 0);\n\t\t\t  usb_reg35: in std_logic_vector(7 downto 0);-- para el canal_6 del ADCdriver\n\t\t\t  usb_reg36: in std_logic_vector(7 downto 0);\n\t\t\t  usb_reg37: in std_logic_vector(7 downto 0);-- para el canal_7 del ADCdriver\n\t\t\t  usb_reg38: in std_logic_vector(7 downto 0);\n\t\t\t  usb_reg39: in std_logic_vector(7 downto 0);-- para el canal_8 del ADCdriver\n\t\t\t  usb_reg40: in std_logic_vector(7 downto 0);\n\t\t\t  usb_reg41: in std_logic_vector(7 downto 0);-- para el canal_9 del ADCdriver\n\t\t\t  usb_reg42: in std_logic_vector(7 downto 0);\n\t\t\t  usb_reg43: in std_logic_vector(7 downto 0);-- para el canal_10 del ADCdriver\n\t\t\t  usb_reg44: in std_logic_vector(7 downto 0)--;  \n\n     usb_reg55 => LVDSByte"
  # "x 100000, que es lo mismo que dividir entre 10^-5ms"
  # "ventana de observación de los scalers en ms"
  # "a 100MHz, que es la velocidad del reloj general de la placa,\ncomo el período es 10^-5ms, para temporizar 50ms (ventana \nque con la tasa de inyección de pulsos de 200KHz contabiliza \n10000 pulsos) el valor hexadecimal de la ventana sería:\n4C4B40"
  n1 = disable-structure shown="Enabled" {
    frame Disabled {
      # "TARJETA 13 TIENE UN POCO MÁS DE \nRUIDO QUE LA 07, PORQUE HAY UN\nPOCO MÁS DE VARIABILIDAD EN LOS \nOFFSET ANALÓGICOS, AUNQUE SALEN\nSIMILARES"
      # "offset sumadores ASIC 373 calculado en tarjeta 13"
      # "offset sumadores ASIC 373 calculado en tarjeta 07"
      n2 = Transpose 2D Array(2D array=dbl[][] [[0.008, -0.023, -0.007], [0.013, -0.019, -0.003], [0.013, -0.019, -0.003], [0.019, -0.013, 0.002], [0.012, -0.019, -0.004], [0.02, -0.011, 0.004], [0.012, -0.019, -0.003]]) -> ()  [unwired: 1 out]
    }
    frame Enabled {
    }
  }
  n3 = Unbundle By Name("Config Test IN") -> ("Config Test"=w66:T5, "Execucion Test.Vasic Actual"=w65:i32)
  n4 = Unbundle By Name("Config Test IN") -> ("Config Test"=w10:T5, "Result"=w15:T7, "Execucion Test.Vasic Actual"=w9:i32)
  n5 = Unbundle By Name("Config Test IN") -> ("Config VGA.Pulse Width"=w60:u16, "Config VGA.Frecuency Pulse"=w59:dbl, "Config VGA.VGA Gain"=w58:u8[], "Config VGA.Real Voltage"=w57:dbl[], "Config VGA.Theoretical Voltage"=w28:dbl[])
  n6 = Unbundle By Name("Config Test IN") -> ("Config HW.Espera acceso FT"=w19:u32, "Config HW.FT_Handle"=w75:u32)
  n7 = Index Array(array=w66, index=w65) -> (element=w64:T6)
  n8 = Index Array(array=w15, index=w9) -> (element=w14:T8)
  n9 = Index Array(array=w10, index=w9) -> (element=w8:T6)
  n10 = Multiply(x=u32 10 ("Ventana"), y=u32 100000 ("Ventana")) -> (x*y=w76:u32)
  n11 = Unbundle By Name(w64) -> ("IBIAS"=w21:bool, "VALUE IBIAS"=w20:u8, "Vin Rate Scan"=w63:i32[], "Limits Rate Scan"=w44:cluster{"High":dbl[], "Low":dbl[]})
  n12 = Unbundle By Name(w14) -> ("Test Offset Analog.V ADDOUT"=w11:dbl[][])
  n13 = Unbundle By Name(w8) -> ("Test offset analog?"=w6:bool)
  n14 = call "VGA_pulso.vi"("Espera acceso USB"=w19, "error in"="Error IN", "Frecuencia pulso (0.2 a 1 Mhz)"=w59, "Patrón (E000)"=w60, "ftHandle_in"=w75) -> ("error out"=w79:errorcluster, "ftHandle_out"=w80:u32)  [unwired: 5 in]
  n15 = call "Scalers_Escribir ventana.vi"("Espera acceso USB"=w19, "error in"=w79, "Ventana"=w76, "ftHandle_in"=w80) -> ("error out"=w77:errorcluster, "ftHandle_out"=w78:u32)  [unwired: 6 in]
  n16 = call "ASIC_reset inicial.vi"("Espera acceso USB"=w19, "error in"=w77, "ftHandle_in"=w78) -> ("error out"=w18:errorcluster, "ftHandle_out"=w74:u32)  [unwired: 7 in]
  n17 = control-ref of="Tab Control"() -> (w31:refnum<vi>)
  n18 = Unbundle By Name(w44) -> ("High"=w43:dbl[], "Low"=w42:dbl[])
  n19 = for {
    tunnel: w63 -> [w85] mode=indexing
    tunnel: w58 -> [w94]
    tunnel: w57 -> [w87]
    tunnel: [w93] -> w29 mode=indexing
    tunnel: [w92] -> w62 mode=indexing
    tunnel: w43 -> [w91]
    tunnel: w42 -> [w90]
    tunnel: [w89] -> w25 mode=indexing
    tunnel: [w88] -> w24 mode=indexing
    tunnel: w28 -> [w86]
    tunnel: [w84] -> w27 mode=indexing
    n20 = Index Array(array=w87, index=w85) -> (element=w92:dbl)
    n21 = Index Array(array=w86, index=w85) -> (element=w84:dbl)
    n22 = Index Array(array=w94, index=w85) -> (element=w93:u8)
    n23 = Index Array(array=w90, index=w85) -> (element=w88:dbl)
    n24 = Index Array(array=w91, index=w85) -> (element=w89:dbl)
  }
  n25 = control-ref of="This VI"() -> (w32:refnum<vi>)
  n26 = call "ASIC_CONFIGURAR IABIAS.vi"("Espera acceso USB"=w19, "error in"=w18, "IBIAS VALUE"=w20, "IBIAS"=w21, "ftHandle_in"=w74) -> ("error out"=w17:errorcluster, "ftHandle_out"=w22:u32)  [unwired: 5 in]
  n27 = for "Canales entrada (7)" {
    N: 7 -> [w108]
    shift-right: [w120] -> w37
    shift-left: w22 -> [w97]
    shift-right: [w119] -> w40
    shift-left: w17 -> [w98]
    tunnel: w19 -> [w96]
    tunnel: w76 -> [w99]
    tunnel: [w118] -> w72 mode=indexing
    tunnel: [w117] -> w71 mode=indexing
    tunnel: w29 -> [w95]
    tunnel: [w116] -> w13 mode=indexing
    tunnel: [w115] -> w56 mode=indexing
    tunnel: w62 -> [w113]
    tunnel: [w112] -> w61 mode=indexing
    tunnel: [w110] -> w48 mode=indexing
    tunnel: [w109] -> w36
    tunnel: w27 -> [w107]
    shift-right: [w105] -> _
    shift-left: 0.0 ("x/y") -> [w106]
    tunnel: w25 -> [w103]
    tunnel: w24 -> [w102]
    shift-right: [w100] -> _
    shift-left: u32 0 ("ms wait IN") -> [w101]
    i -> [w114]
    stop <- w104 stop-if-true
    n28 = To Unsigned Byte Integer(number=w114) -> (unsigned 8bit integer=w111:u8)
    n29 = for "Sumadores (3)" {
      N: 3 -> [w132]
      tunnel: w96 -> [w145]
      tunnel: w99 -> [w146]
      shift-right: [w143] -> w120
      shift-left: w97 -> [w149]
      shift-right: [w142] -> w119
      shift-left: w98 -> [w148]
      tunnel: [w141] -> w118 mode=indexing
      tunnel: [w140] -> w117 mode=indexing
      tunnel: [w139] -> w116 mode=indexing
      tunnel: [w138] -> w115 mode=indexing
      tunnel: w111 -> [w137]
      tunnel: w113 -> [w136]
      tunnel: [w135] -> w112 mode=indexing
      tunnel: [w134] -> w110 mode=indexing
      tunnel: [w133] -> w109
      tunnel: w108 -> [w131]
      tunnel: w107 -> [w130]
      shift-right: [w128] -> w105
      shift-left: w106 -> [w129]
      tunnel: [w127] -> w104
      tunnel: w103 -> [w126]
      tunnel: w102 -> [w125]
      shift-right: [w123] -> w100
      shift-left: w101 -> [w124]
      tunnel: w95 -> [w122]
      i -> [w147]
      stop <- w127 stop-if-true
      n30 = To Unsigned Byte Integer(number=w147) -> (unsigned 8bit integer=w144:u8)
      n31 = for "Tensiones asic" {
        N -> [w182]
        tunnel: w144 -> [w178]
        tunnel: w146 -> [w154]
        tunnel: w145 -> [w150]
        shift-right: [w186] -> w142
        shift-left: w148 -> [w155]
        shift-right: [w187] -> w143
        shift-left: w149 -> [w156]
        tunnel: [w189] -> w141 mode=indexing
        tunnel: [w188] -> w140 mode=indexing
        tunnel: [w171] -> w139 mode=indexing
        tunnel: [w170] -> w138 mode=indexing
        tunnel: w137 -> [w183]
        tunnel: w136 -> [w179] mode=indexing
        tunnel: [w185] -> w135 mode=indexing
        tunnel: [w184] -> w134 mode=indexing
        tunnel: [w162] -> w133
        tunnel: w132 -> [w181]
        tunnel: w131 -> [w180]
        tunnel: w130 -> [w176] mode=indexing
        shift-right: [w174] -> w128
        shift-left: w129 -> [w175]
        tunnel: [w167] -> w127
        tunnel: w126 -> [w173] mode=indexing
        tunnel: w125 -> [w172] mode=indexing
        shift-right: [w166] -> w123
        shift-left: w124 -> [w168]
        tunnel: w122 -> [w153] mode=indexing
        i -> [w177]
        stop <- w167 stop-if-true
        n32 = call "ADC_inicialización Setup-Averaging.vi"("ftHandle_in 2"=w156, "Espera acceso USB"=w150, "Reset (T=reset)"=TRUE, "Registro Setup (0x6800)"=u16 26624, "Registro Averaging (0x3200)"=u16 8192 ("Registro Setup (0x6800)"), "error in 2"=w155) -> ("ftHandle_out"=w161:u32, "error out"=w160:errorcluster)  [unwired: 8 in]
        n33 = call "VGA_ganancia.vi"("Espera acceso USB"=w150, "error in 2"=w160, "Ganancia"=w153, "ftHandle_in 2"=w161) -> ("error out 2"=w152:errorcluster, "ftHandle_out 2"=w151:u32)  [unwired: 6 in]
        n34 = for "Reintentos" {
          N: 3 -> [_]
          tunnel: [w197] -> w189
          tunnel: [w196] -> w188
          tunnel: w154 -> [w204]
          tunnel: w151 -> [w242]
          tunnel: [w239] -> w187
          tunnel: [w236] -> w185
          tunnel: [w235] -> w184
          tunnel: w150 -> [w203]
          tunnel: w183 -> [w191]
          tunnel: w182 -> [w233]
          tunnel: w181 -> [w232]
          tunnel: w180 -> [w231]
          tunnel: w179 -> [w228]
          tunnel: w178 -> [w192]
          tunnel: w177 -> [w226]
          tunnel: w176 -> [w223]
          tunnel: [w211] -> w167
          tunnel: w173 -> [w217]
          tunnel: w172 -> [w216]
          tunnel: [w215] -> w171
          tunnel: [w214] -> w170
          shift-right: [w238] -> w186
          shift-left: w152 -> [w243]
          tunnel: w175 -> [w220]
          tunnel: [w218] -> w174
          shift-right: [w193] -> w165
          shift-left: w168 -> [w193]
          tunnel: [w208] -> w163
          tunnel: [w195] -> w162
          i -> [w207]
          stop <- w210 stop-if-true
          w205 = u32 3  # ERRORES MAXIMOS
          w245 = TRUE  # Reset (T=reset)
          n35 = Compound Arithmetic op=MULTIPLY(w233, w232, w231) -> (w230:i32)
          n36 = Divide(x=100.0, y=w230) -> (x/y=w219:dbl)
          n37 = To Unsigned Byte Integer(number=w226) -> (unsigned 8bit integer=w190:u8)
          n38 = Add(x=w219, y=w220) -> (x+y=w218:dbl)
          n39 = local write "%"(w218) -> ()
          n40 = local write "B"(w218) -> ()
          n41 = call "ASIC_Selecor canal Sumador.vi"("Espera acceso USB"=w203, "error in"=w243, "Sumador"=w190, "Canal"=w192, "ftHandle_in"=w242) -> ("error out"=w241:errorcluster, "ftHandle_out"=w240:u32)  [unwired: 4 in, 1 out]
          n42 = Index Array(array=string[] ["A", "B", "C"], index=w192) -> (element=w225:string)
          n43 = call "ADC_inicialización Setup-Averaging.vi"("ftHandle_in 2"=w240, "Espera acceso USB"=w203, "Reset (T=reset)"=w245, "Registro Setup (0x6800)"=u16 26624, "Registro Averaging (0x3200)"=u16 8192 ("Registro Setup (0x6800)"), "error in 2"=w241) -> ("ftHandle_out"=w202:u32, "error out"=w201:errorcluster)  [unwired: 8 in]
          n44 = call "Rate scan.vi"("T Ventana"=w204, "Espera acceso USB"=w203, "error in 2"=w201, "Valor buscado scalers (5000)"=u16 5000 ("Valor buscado scalers"), "Sumador"=w190, "ftHandle_in 2"=w202) -> ("error out 2"=w199:errorcluster, "DAC\nTH3,TH4,TH5"=w196:u16, "DAC\nTH0,TH1,TH2"=w197:u16, "ftHandle_out 2"=w200:u32, "Scaler 1"=w236:u16)  [unwired: 1 in]
          "DAC TH0,TH1,TH2" <- w197
          "DAC TH3,TH4,TH5" <- w196
          n45 = Bundle(cluster=T1 {"Sumador"=0, "Canal"=0, "Tension"=0, "Tension Real"=0.0}, "Sumador"=w192, "Canal"=w191, "Tension"=w190, "Tension Real"=w228) -> (w235:T1)
          "Reference" <- w235
          n46 = Increment(x=w191) -> (x+1=w222:u8)
          n47 = case shown="False" FALSE {
            tunnel: [w255 w266] -> w239
            tunnel: [w249 w265] -> w238
            tunnel: [w247 w264] -> w215
            tunnel: [w248 w263] -> w214
            tunnel: w203 -> [w246 w256]
            tunnel: w190 -> [w253 w262]
            tunnel: w200 -> [w254 w261]
            tunnel: w199 -> [w250 w260]
            tunnel: w197 -> [w252 w259]
            tunnel: w196 -> [w251 w258]
            tunnel: [w246 w256] -> w195
            frame False {
              n48 = call "ASIC_WRITE THX THX3 READ ADC.vi"("ftHandle_in"=w254, "Sumador"=w253, "THX"=w252, "THX+3"=w251, "error in"=w250, "Espera acceso USB 2"=w246) -> ("ftHandle_out"=w255:u32, "HLTHx"=w247:dbl, "LLTHx"=w248:dbl, "error out"=w249:errorcluster)  [unwired: 10 in]
            }
            frame True {
              n49 = call "ADC_READ VHLTHx VLLTHx.vi"("ftHandle_out 2"=w261, "Sumador"=w262, "referenciar"=TRUE, "ref DAC\nTH0,TH1,TH2"=w259, "ref DAC\nTH3,TH4,TH5"=w258, "error out 2"=w260, "Espera acceso FT"=w256) -> ("ftHandle_out"=w266:u32, "HLTHx"=w264:dbl, "LLTHx"=w263:dbl, "error out"=w265:errorcluster)  [unwired: 8 in, 1 out]
            }
          }
          "HLTHx" <- w215
          "LLTHx" <- w214
          n50 = call "Barra puntos.vi"("#N"=w207) -> ("String"=w206:string)  [unwired: 8 in]
          n51 = Format Into String(format string="Vin %,;%1.4fV Channel %d Adder %s\n%sTotal Errors: %d%s", w223, w222, w225, w206, w193, w206) -> (resulting string=w224:string)  [unwired: 2 in, 1 out]
          n52 = local write "Indicador"(w224) -> ()
          n53 = global read "Global.Salir Ya.vi" "Cancel"() -> (w211:bool)
          n54 = In Range and Coerce(upper limit=w217, x=w215, lower limit=w216) -> (In Range?=w212:bool)  [unwired: 1 out]
          n55 = In Range and Coerce(upper limit=w217, x=w214, lower limit=w216) -> (In Range?=w213:bool)  [unwired: 1 out]
          n56 = Greater?(x=w193, y=w205) -> (0:w209:bool)
          n57 = And(x=w212, y=w213) -> (x .and. y?=w208:bool)
          n58 = Compound Arithmetic op=OR(w208, w211, w209) -> (w210:bool)
        }
        n59 = Increment(x=w165) -> (x+1=w164:u32)
        n60 = Select(t=w165, s=w163, f=w164) -> (s? t:f=w166:u32)
      }
      "Array" <- w139
      "Array 2" <- w138
    }
  }
  "DAC TH0,TH1,TH2" <- w72
  "DAC TH3,TH4,TH5" <- w71
  "Volt HLTH (salida A)" <- w13
  "Volt LLTH (salida B)" <- w56
  n61 = property class="VI"(reference=w32, "Front Panel.ShowMenuBar"=w35, "TB.Visible"=w35, "Front Panel.TitleBarVis"=TRUE ("Front Panel Window:Title Bar Visible"), "Front Panel.Title"="TEST ASIC. Rate Scan" ("Front Panel Window:Title")) -> ("Panel"=w3:refnum<vi>)  [unwired: 1 in, 2 out]
  n62 = disable-structure shown="Enabled" {
    disable-tunnel: w32 -> [w269 _]
    disable-tunnel: w31 -> [w268 _]
    disable-tunnel: "Error IN" -> [w267 _]
    frame Disabled {
      n63 = call "WINDOWS.AUTO SIZE.vi"("Error In"=w267, "TAB.AutoAjuste"=w268, "This VI"=w269) -> ()  [unwired: 4 in, 1 out]
    }
    frame Enabled {
    }
  }
  n64 = property class="Pnl"(reference=w3) -> ("Panes[]"=w2:refnum<vi>[])  [unwired: 1 in, 2 out]
  n65 = for {
    tunnel: w2 -> [w272] mode=indexing
    tunnel: w1 -> [w271]
    tunnel: w1 -> [w270]
    n66 = property class="Pane"(reference=w272, "VertScrollbarVisibility"=w271, "HorizScrollbarVisibility"=w270) -> ()  [unwired: 1 in, 2 out]
  }
  n67 = Delete From Array(array=w11, index (row)=7) -> (array with subset deleted=w7:dbl[][])  [unwired: 2 in, 1 out]
  n68 = for {
    tunnel: w13 -> [w277] mode=indexing
    tunnel: w56 -> [w279] mode=indexing
    tunnel: [w283] -> w45 mode=indexing
    tunnel: [w284] -> w46 mode=indexing
    tunnel: w25 -> [w282] mode=indexing
    tunnel: w24 -> [w281] mode=indexing
    tunnel: w7 -> [w274]
    tunnel: w6 -> [w276]
    n69 = Subtract "array=0 no offset"(x=w277, y=w277) -> (x-y=w275:dbl[][])
    n70 = Select(t=w274, s=w276, f=w275) -> (s? t:f=w273:dbl[][])
    n71 = Subtract(x=w277, y=w273) -> (x-y=w280:dbl[][])
    n72 = Subtract(x=w279, y=w273) -> (x-y=w278:dbl[][])
    n73 = In Range and Coerce(upper limit=w282, x=w280, lower limit=w281) -> (In Range?=w283:bool[][])  [unwired: 1 out]
    n74 = In Range and Coerce(upper limit=w282, x=w278, lower limit=w281) -> (In Range?=w284:bool[][])  [unwired: 1 out]
  }
  "Comparation HLTH" <- w45
  "Comparation LLTH" <- w46
  n75 = Unbundle By Name("Config Test IN") -> ("Result"=w69:T7, "Execucion Test.Vasic Actual"=w68:i32)
  n76 = Array Size(array=w13) -> (size(s)=w55:i32[])
  n77 = Index Array(array=w55) -> (element #1=w54:i32, element #2=w53:i32, element #3=w52:i32)  [unwired: 3 in]
  n78 = Index Array(array=w69, index=w68) -> (element=w73:T8)
  n79 = Initialize Array(TRUE, w54, w53, w52) -> (w41:bool[][][])
  n80 = Equal?(x=w45, y=w41) -> (x = y?=w50:bool)
  n81 = Equal?(x=w46, y=w41) -> (x = y?=w49:bool)
  n82 = call "ASIC_reset inicial.vi"("Espera acceso USB"=w36, "error in"=w40, "ftHandle_in"=w37) -> ("error out"=→"Error OUT":errorcluster, "ftHandle_out"=w38:u32)  [unwired: 7 in]
  n83 = And(x=w50, y=w49) -> (x .and. y?=w47:bool)
  "Rate scan all ok" <- w47
  n84 = Bundle By Name(cluster=w73, "Test Rate Scan.Scaler 0"=w61, "Test Rate Scan.DAC TH0,TH1,TH2"=w72, "Test Rate Scan.DAC TH3,TH4,TH5"=w71, "Test Rate Scan.Volt HLTH"=w13, "Test Rate Scan.Volt LLTH"=w56, "Test Rate Scan.Rate HLTH OK"=w45, "Test Rate Scan.Rate LLTH 2 OK"=w46, "Test Rate Scan.Rate Scan OK"=w47, "Test Rate Scan.Ref"=w48) -> (w70:T8)
  n85 = Insert Into Array(array=w69, index=w68, new element=w70) -> (w67:T7)
  n86 = Bundle By Name(cluster="Config Test IN", "Result"=w67, "Config HW.FT_Handle"=w38) -> (w5:T2)
  "Config Test OUT" <- w5
  n87 = flat-sequence {
    tunnel: w5 -> [_]
    frame #0 {
      n88 = control-ref of="This VI"() -> (w285:refnum<vi>)
      n89 = invoke class="VI" method="FP.Close"(reference=w285) -> ()  [unwired: 2 in, 3 out]
    }
  }
